vi "niFpga wdp fft 4wire fifo dummy.vi"(8 "read?":bool, 9 "write?":bool, 10 "data in im":fxp<+/-,8,1>[](array[numeric])=[0.0, 0.0], 11 "data in re":fxp<+/-,8,1>[](array[numeric])=[0.0, 0.0]) -> (2 "data out im":fxp<+/-,8,1>[](array[numeric]), 3 "data out re":fxp<+/-,8,1>[](array[numeric]))   [LabVIEW 2017]
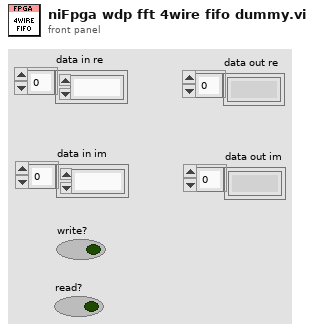
[diagram p1: front panel]
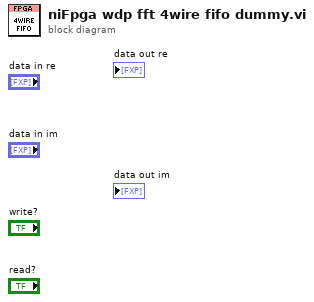
[diagram p0: block diagram]
diagram:
